vi "reorder lists.vi"(11 "sorted list":T1) -> (3 "ordered list":string[](array[string]))   [LabVIEW 2013, in "tag bus.lvlib" / "binary search.lvlib"]
doc: "Converts a set of sorted strings into an array of strings sorted by index."
uses:
  binary search.lvlib
  sorted list.ctl
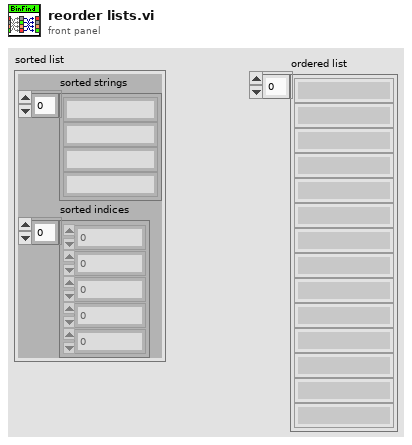
[diagram p1: front panel]
types:
  T1 = typedef "tag bus.lvlib/binary search.lvlib/sorted list.ctl" = cluster{"sorted strings":string[], "sorted indices":i32[]}
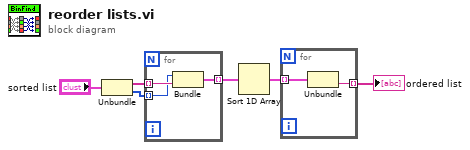
[diagram p0: block diagram]
diagram:
  n1 = Unbundle("sorted list") -> ("sorted strings"=w5:string[], "sorted indices"=w4:i32[])
  n2 = for {
    tunnel: w5 -> [w9] mode=indexing
    tunnel: w4 -> [w8] mode=indexing
    tunnel: [w7] -> w3 mode=indexing
    n3 = Bundle("Numeric"=w8, "String"=w9) -> (w7:cluster{"Numeric":i32, "String":string})  [unwired: 1 in]
  }
  n4 = Sort 1D Array(array=w3) -> (sorted array=w2:cluster{"Numeric":i32, "String":string}[])
  n5 = for {
    tunnel: w2 -> [w11] mode=indexing
    tunnel: [w10] -> w1 mode=indexing
    n6 = Unbundle(w11) -> ("String"=w10:string)  [unwired: 1 out]
  }
  "ordered list" <- w1
